vi "Experiment02.vi"() -> ()   [LabVIEW 2009]
uses:
  <vilib>/imath/engines/lvmath2/RunTimeEngine/ErrorHandling/NIMS_Finalize Error.vi
  <vilib>/imath/engines/lvmath2/RunTimeEngine/Parser/MC_Version.vi
  <vilib>/imath/engines/lvmath2/RunTimeEngine/NodeEndStatement/NIMS_NodeEndStatement_Output.vi
  <instcachedir>/0/NIMS_NodeEndStatement_Output_B70DDD75627E4997AAE11E9955EDAA25.lvgen/NIMS_NodeEndStatement_Output_B70DDD75627E4997AAE11E9955EDAA25_003.vi
  <instcachedir>/0/NIMS_NodeEndStatement_Output_B70DDD75627E4997AAE11E9955EDAA25.lvgen/NIMS_NodeEndStatement_Output_B70DDD75627E4997AAE11E9955EDAA25_002.vi
  <vilib>/imath/engines/lvmath/Functions/Error Handling/MergeErrorsWrapper.vi
  <instcachedir>/0/NIMS_NodeEndStatement_Output_B70DDD75627E4997AAE11E9955EDAA25.lvgen/NIMS_NodeEndStatement_Output_B70DDD75627E4997AAE11E9955EDAA25_001.vi
  <vilib>/imath/engines/lvmath2/RunTimeEngine/Managers/WorkSpace/UID Generator.vi
  <vilib>/imath/engines/lvmath/Functions/Error Handling/error.ctl
  <instcachedir>/0/NIMS_NodeEndStatement_Output_B70DDD75627E4997AAE11E9955EDAA25.lvgen/NIMS_NodeEndStatement_Output_B70DDD75627E4997AAE11E9955EDAA25_000.vi
  <vilib>/imath/engines/lvmath2/RunTimeEngine/Managers/SymbolTable/Clear UID.vi
  <vilib>/imath/engines/lvmath2/RunTimeEngine/VariableToken/NIMS_VariableToken_CondDefined.vi
  <instcachedir>/0/NIMS_VariableToken_CondDefined_5641E79000FB4D628475532441475385.lvgen/NIMS_VariableToken_CondDefined_5641E79000FB4D628475532441475385_001.vi
  <vilib>/imath/engines/lvmath/Functions/Error Handling/MC_Mask_Errors.vi
  <vilib>/imath/engines/lvmath2/RunTimeEngine/BuiltInFunctions/rem/NIMS_rem_no checks.vi
  <instcachedir>/0/NIMS_rem_no checks_4CC9B305AB7E42EF90AFC4973FB32F8D.lvgen/NIMS_rem_no checks_4CC9B305AB7E42EF90AFC4973FB32F8D_000.vi
  <vilib>/imath/engines/lvmath2/RunTimeEngine/BuiltInFunctions/uint32/NIMS_uint32(real).vi
  <instcachedir>/0/NIMS_uint32(real)_FDC83D68D45943DDB8F3F934FF8A712F.lvgen/NIMS_uint32(real)_FDC83D68D45943DDB8F3F934FF8A712F_000.vi
  <vilib>/imath/engines/lvmath2/RunTimeEngine/BuiltInFunctions/double/NIMS_double.vi
  <instcachedir>/0/NIMS_double_2CE444F3CE4146B199A482FE12545E45.lvgen/NIMS_double_2CE444F3CE4146B199A482FE12545E45_000.vi
  <vilib>/imath/engines/lvmath2/RunTimeEngine/RangeToken/NIMS_Range.vi
  <instcachedir>/0/NIMS_Range_6D647EC16A744C98B5DE1D649A2D648D.lvgen/NIMS_Range_6D647EC16A744C98B5DE1D649A2D648D_001.vi
  <vilib>/imath/engines/lvmath2/RunTimeEngine/BuiltInFunctions/length/NIMS_length(GV).vi
  <instcachedir>/0/NIMS_length(GV)_7D6E94E728E145E68721C53861296D96.lvgen/NIMS_length(GV)_7D6E94E728E145E68721C53861296D96_000.vi
  <instcachedir>/0/NIMS_Range_6D647EC16A744C98B5DE1D649A2D648D.lvgen/NIMS_Range_6D647EC16A744C98B5DE1D649A2D648D_000.vi
  <vilib>/imathl/engines/lvmath/Functions/Error Handling/Create Error.vi
  <vilib>/imath/engines/lvmath2/RunTimeEngine/ReplaceToken/NIMS_Replace - V(S)=S.vi
  <instcachedir>/0/NIMS_Replace - V(S)=S_670A9E0533664C1D848C8E58B3321B6A.lvgen/NIMS_Replace - V(S)=S_670A9E0533664C1D848C8E58B3321B6A_002.vi
  <vilib>/imath/engines/lvmath2/RunTimeEngine/ReplaceToken/NIMS_Replace - Size Check _(_)=S.vi
  <instcachedir>/0/NIMS_Replace - Size Check _(_)=S_8596181D73404097BAB9CBB006194BB0.lvgen/NIMS_Replace - Size Check _(_)=S_8596181D73404097BAB9CBB006194BB0_002.vi
  <vilib>/imath/engines/lvmath2/RunTimeEngine/ReplaceToken/NIMS_Replace - Check Linear.vi
  <instcachedir>/0/NIMS_Replace - Check Linear_9243CBB174894FF6977027453DA6955E.lvgen/NIMS_Replace - Check Linear_9243CBB174894FF6977027453DA6955E_002.vi
  <vilib>/imath/engines/lvmath2/RunTimeEngine/VariableToken/NIMS_VariableToken_CondDefinedDefinedByReplace.vi
  <instcachedir>/0/NIMS_VariableToken_CondDefinedDefinedByReplace_D162CFFC24174562A9FEA619A91E1A56.lvgen/NIMS_VariableToken_CondDefinedDefinedByReplace_D162CFFC24174562A9FEA619A91E1A56_002.vi
  <vilib>/imath/engines/lvmath2/RunTimeEngine/CommandStatement/MC_CommandStatement_break.vi
  <vilib>/imath/engines/lvmath2/RunTimeEngine/LocalVariableDefStatement/MC_LocalVariableDefStatement_Display.vi
  <vilib>/imath/engines/lvmath2/RunTimeEngine/RunTimeType/NIMS_RunTimeType_From StrictType (excl LVString).vi
  <vilib>/imath/engines/lvmath2/RunTimeEngine/ArithmeticOperatorToken/NIMS_ArithmeticOperator_times.vi
  <instcachedir>/0/NIMS_ArithmeticOperator_times_3987BC660D7947CD8628C10658A43225.lvgen/NIMS_ArithmeticOperator_times_3987BC660D7947CD8628C10658A43225_001.vi
  <instcachedir>/0/NIMS_ArithmeticOperator_times_3987BC660D7947CD8628C10658A43225.lvgen/NIMS_ArithmeticOperator_times_3987BC660D7947CD8628C10658A43225_000.vi
  <vilib>/imath/engines/lvmath2/RunTimeEngine/VariableToken/Read/NIMS_Get Elements - RV(_) - Check.vi
  <instcachedir>/0/NIMS_Get Elements - RV(_) - Check_60F12861D0564803969A5D0D0D1716CD.lvgen/NIMS_Get Elements - RV(_) - Check_60F12861D0564803969A5D0D0D1716CD_000.vi
  <instcachedir>/0/NIMS_VariableToken_CondDefined_5641E79000FB4D628475532441475385.lvgen/NIMS_VariableToken_CondDefined_5641E79000FB4D628475532441475385_000.vi
  <vilib>/imath/engines/lvmath2/RunTimeEngine/BuiltInFunctions/abs/NIMS_abs(signed).vi
  <instcachedir>/0/NIMS_abs(signed)_C4FCB8E6058B49B797C7C8D53CA5F6EC.lvgen/NIMS_abs(signed)_C4FCB8E6058B49B797C7C8D53CA5F6EC_000.vi
  <instcachedir>/0/NIMS_Replace - V(S)=S_670A9E0533664C1D848C8E58B3321B6A.lvgen/NIMS_Replace - V(S)=S_670A9E0533664C1D848C8E58B3321B6A_001.vi
  <instcachedir>/0/NIMS_Replace - Size Check _(_)=S_8596181D73404097BAB9CBB006194BB0.lvgen/NIMS_Replace - Size Check _(_)=S_8596181D73404097BAB9CBB006194BB0_001.vi
  <instcachedir>/0/NIMS_Replace - Check Linear_9243CBB174894FF6977027453DA6955E.lvgen/NIMS_Replace - Check Linear_9243CBB174894FF6977027453DA6955E_001.vi
  <instcachedir>/0/NIMS_VariableToken_CondDefinedDefinedByReplace_D162CFFC24174562A9FEA619A91E1A56.lvgen/NIMS_VariableToken_CondDefinedDefinedByReplace_D162CFFC24174562A9FEA619A91E1A56_001.vi
  <instcachedir>/0/NIMS_Replace - V(S)=S_670A9E0533664C1D848C8E58B3321B6A.lvgen/NIMS_Replace - V(S)=S_670A9E0533664C1D848C8E58B3321B6A_000.vi
  <instcachedir>/0/NIMS_Replace - Size Check _(_)=S_8596181D73404097BAB9CBB006194BB0.lvgen/NIMS_Replace - Size Check _(_)=S_8596181D73404097BAB9CBB006194BB0_000.vi
  <instcachedir>/0/NIMS_Replace - Check Linear_9243CBB174894FF6977027453DA6955E.lvgen/NIMS_Replace - Check Linear_9243CBB174894FF6977027453DA6955E_000.vi
  <instcachedir>/0/NIMS_VariableToken_CondDefinedDefinedByReplace_D162CFFC24174562A9FEA619A91E1A56.lvgen/NIMS_VariableToken_CondDefinedDefinedByReplace_D162CFFC24174562A9FEA619A91E1A56_000.vi
  <vilib>/imath/engines/lvmath2/RunTimeEngine/BuiltInFunctions/imag/NIMS_imag(Complex).vi
  <instcachedir>/0/NIMS_imag(Complex)_D35A2F120E254B34824E500A22AD8EA0.lvgen/NIMS_imag(Complex)_D35A2F120E254B34824E500A22AD8EA0_000.vi
  <vilib>/imath/engines/lvmath2/RunTimeEngine/Managers/SymbolTable/NIMS_WorkSpace.lvlib
panel:
  out "Current VI path 12":string
  out "New Path for Picture 12":string
  out "Part Stripped 12":string
  out "Stripped Path 12":string
  out "Current VI path 11":string
  out "New Path for Picture 11":string
  out "Part Stripped 11":string
  out "Stripped Path 11":string
  out "Current VI path 10":string
  out "New Path for Picture 10":string
  out "Part Stripped 10":string
  out "Stripped Path 10":string
  out "Current VI path 9":string
  out "New Path for Picture 9":string
  out "Part Stripped 9":string
  out "Stripped Path 9":string
  out "Current VI path 8":string
  out "New Path for Picture 8":string
  out "Part Stripped 8":string
  out "Stripped Path 8":string
  out "Current VI path 7":string
  out "New Path for Picture 7":string
  out "Part Stripped 7":string
  out "Stripped Path 7":string
  out "Current VI path 6":string
  out "New Path for Picture 6":string
  out "Part Stripped 6":string
  out "Stripped Path 6":string
  out "Current VI path 5":string
  out "New Path for Picture 5":string
  out "Part Stripped 5":string
  out "Stripped Path 5":string
  out "Current VI path 4":string
  out "New Path for Picture 4":string
  out "Part Stripped 4":string
  out "Stripped Path 4":string
  out "Current VI path 3":string
  out "New Path for Picture 3":string
  out "Part Stripped 3":string
  out "Stripped Path 3":string
  out "Current VI path 2":string
  out "New Path for Picture 2":string
  out "Part Stripped 2":string
  out "Stripped Path 2":string
  out "Current VI path":string
  out "New Path for Picture":string
  out "Part Stripped":string
  out "Stripped Path":string
  out "error out":errorcluster
  in  "HELP FOR VSWR":bool
  out "error out":errorcluster
  out "?":errorcluster
  in  "VSWR Value of Unknown Impedance":bool
  out "?":errorcluster
  out "VSWR Meter":dbl(knob) caption="Meter" scale=500.0..1.0 scale format="%#_10g"
  in  "?":enum32{"LOADS"}(tab)
  in  "Type of Loads":T1(radio)
  out "Resistance 2":dbl
  out "Reactance":dbl
  in  "Resistance":dbl(slide) scale=0.0..1000.0
  in  "Reluctance":dbl(slide) scale=0.0..1000.0
  out "?":errorcluster
  in  "HELP FOR LOADS":bool
  out "error out":errorcluster
  in  "?":enum32{"SLOTTED LINE(VOLTAGE)"}(tab)
  out "?":dbl[](graph)
  in  "Slide":dbl(slide) scale=0.0..0.3
  out "Voltage":dbl
  out "Distance(Meter)":dbl
  out "Characteristic Impedance":dbl
  in  "Short Circuited              Load":bool
  out "?":errorcluster
  in  "First Minima from Load(Unknown Impedance)":bool
  out "?":dbl
  in  "First Minima from Load(Short Circuited)":bool
  in  "Second Minima from Load(Short Circuited)":bool
  out "?":dbl
  in  "HELP FOR SLOTTED LINE":bool
  out "?":dbl
  in  "?":enum32{"ATTENUATOR"}(tab)
  out "?":dbl[](graph)
  in  "Set the value of attenuation in dB":dbl(slide) scale=0.0..100.0
  out "?":errorcluster
  in  "HELP FOR ATTENUATOR":bool
  out "error out":errorcluster
  in  "?":enum32{"ISOLATOR"}(tab)
  out "?":dbl[](graph)
  in  "?":bool
  out "?":errorcluster
  in  "HELP FOR ISOLATOR":bool
  out "error out":errorcluster
  in  "?":enum32{"MODULATOR"}(tab)
  out "?":dbl[](graph)
  in  "Modulating Frequency(KHz)":dbl(slide) scale=0.5..1.5
  out "?":errorcluster
  in  "HELP FOR MODULATOR":bool
  out "error out":errorcluster
  in  "?":enum32{"SOURCE"}(tab)
  out "?":dbl[](graph)
  in  "Frequency of carrier wave(GHz)":dbl(slide) scale=8.0..15.0
  in  "Voltage 3":dbl(knob) scale=0.0..20.0 scale format="%#_10g"
  out "?":errorcluster
  in  "HELP FOR SOURCE":bool
  out "error out":errorcluster
  out "?":errorcluster
  out "Reactance of Unknown Impedance":dbl
  out "Resistance of Unknown Impedance":dbl
  in  "Value of Unknown Impedance":bool
  # "Backward Direction"
  # "Forward direction"
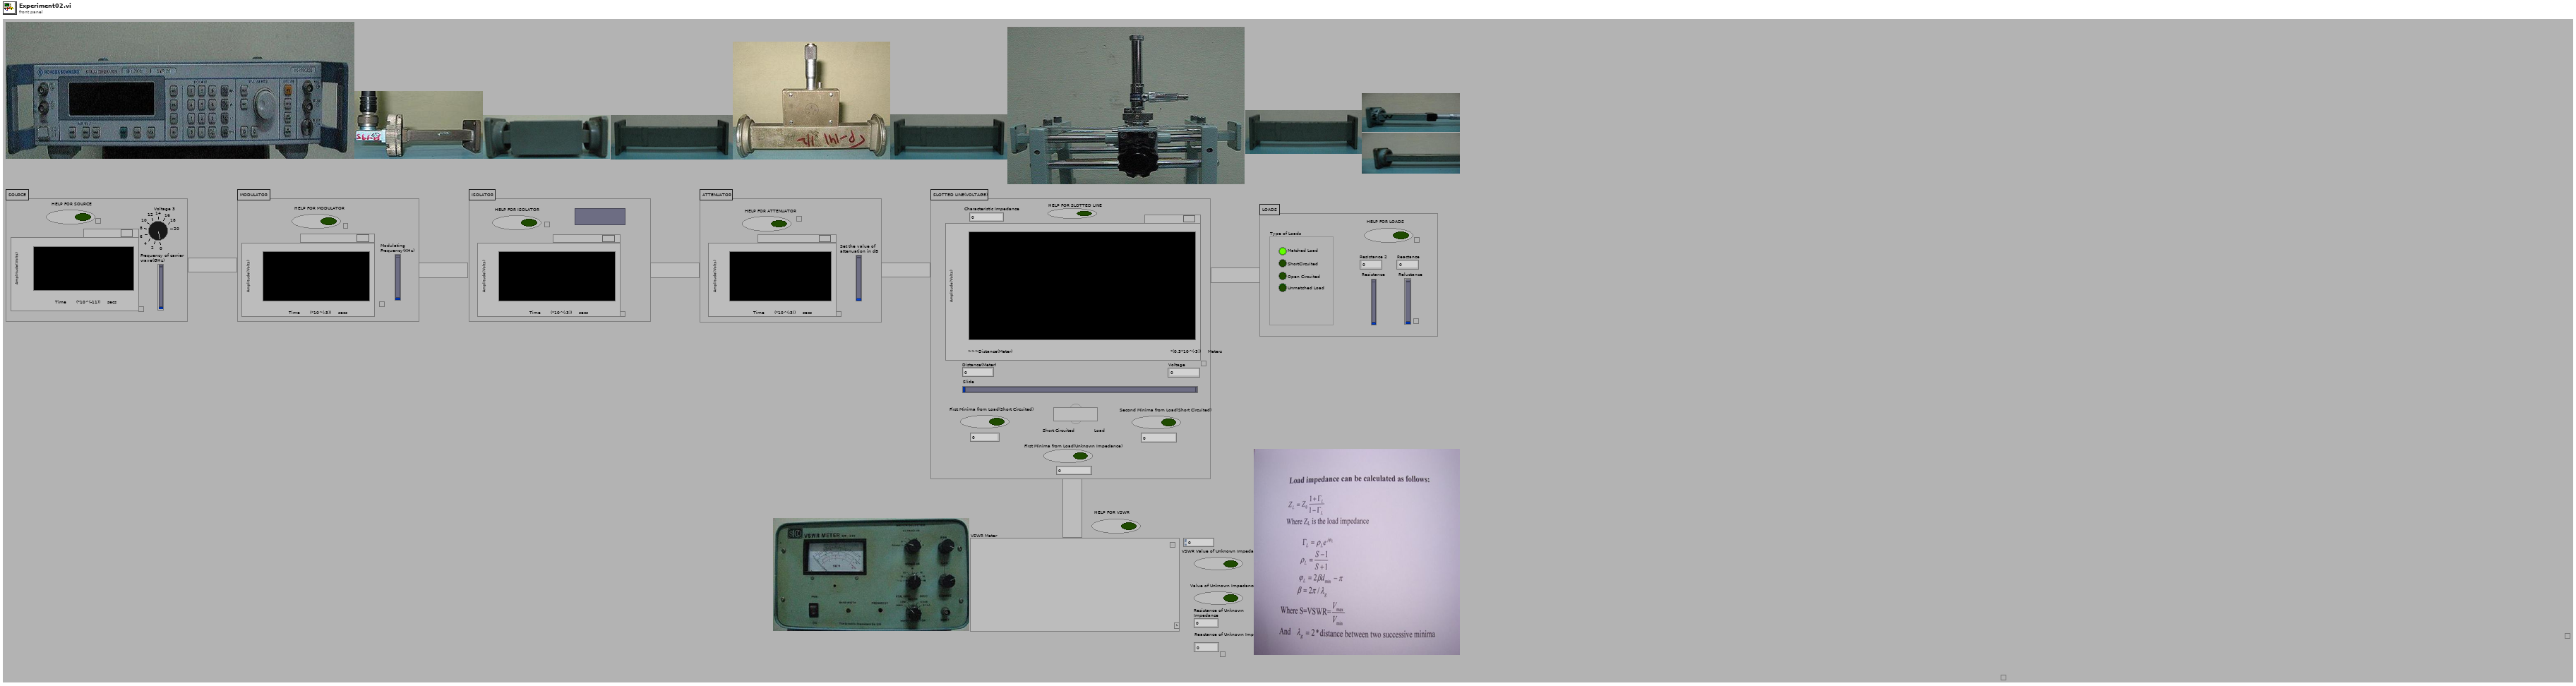
[diagram p1: front panel]
types:
  T1 = enum32{"Matched Load", "ShortCircuited", "Open Circuited", "Unmatched Load"}
  T2 = typedef "imagedata.ctl" = cluster{"image type":i32, "image depth":i32, "image":u8[], "mask":u8[], "colors":u32[], "Rectangle":cluster{"left":i16, "top":i16, "right":i16, "bottom":i16}}
  T3 = typedef "error.ctl" = enum16{"No Error", "Problem", "Unused002", "Incorrect number of parameters", "Function not defined for non-numeric types", "Unused005", "Function only defined for character arrays", "Function not defined for boolean, character, or single precision", "Function not defined for complex types", "Not a valid operation", "Inputs must be scalar", "Input matrices are not the same size", "Unused012", "Input matrices must be nonnegative integers of the same type", "Arguments must be non-negative integers less than bitmax", "Number to complement must be less than 2^N", "Bit to get is outside range", "Bit to set is outside range", "Input must be real type ", "At least one parameter must be scalar", "Unused020", "Function not defined for\nhigher dimensional matrices.", "Invalid attributes", "Wrong Type of Input Arguments", "Wrong Argument Option", "Unused025", "Indices must be real positive integers", "Unused027", "Number of elements must be the same for indices and values", "Unused029", "Cannot resize a 2D matrix with a linear index", "Unknown variable or symbol", "Indices out of range", "Empty matrix deletion can not be used with two indices", "Number of rows and columns must be the same for indices and values.", "Complex cannot be converted to Boolean", "Char cannot be converted to Boolean", "int64 cannot be converted to Boolean", "uint64 cannot be converted to Boolean", "Unused039", "Unused040", "All rows must have the same number of columns", "Incompatible types", "Invalid matrix dimensions", "Dimension must be 1 or 2", "Base must be an integer between 2 and 36", "Invalid input", "Square matrix required", "Function 'timerstart' must be called before 'timerstop'", "Arguments must be positive real", "Step must not be zero", "Wrong number of input arguments", "Wrong number of output arguments", "Unused053", "Input scalar must be >= 0", "Input scalar must be positive", "Input scalar must not be 0", "Input scalar must be in range [0,1]", "Unused058", "Input must be a vector", "Unused060", "Empty vector error", "All elements must be in domain [-1,1]", "All real elements of input vector must be >= 0", "All elements of input vector must be positive", "Values of input vectors are not compatible", "Unused066", "Input vector must be an increasing vector", "Unused068", "Unused069", "Lenths of two input vectors are not compatible", "Unused071", "Empty matrix error", "Unused073", "Unused074", "Unused075", "Unused076", "Unused077", "Size of input matrix is incompatible with input size", "Invalid format specifier", "Unused080", "Unused081", "Unused082", "Unused083", "Unused084", "Unused085", "RunTime: MathScript could not be compiled", "Unknown function", "Only scalars and strings supported", "Unused089", "Unused090", "Range is too large", "End used without variable", "Function not available (RTE)", "Custom user error", "Arguments must be integers less than bitmax", "Shared library not found", "Header file not found", "Shared library already loaded", "Shared library not loaded", "Shared library function not found", "Shared library string return problem", "Problem calling shared library function", "Problem loading shared library from OS", "Problem parsing shared library header file", "Shared library incompatible types", "Shared library unsupported return type", "Shared library function not exported", "Shared library unsupported input type", "Problem unloading shared library from OS", "Function only available from UI", "Invalid function specified in argument", "An internal error has occurred", "Invalid object", "Invalid property", "Read-only property", "A break command has occurred", "A continue command has occurred", "A return command has occurred", "ode: times parameter invalid", "Unused120", "Function not found in file", "Reserved keyword cannot be defined as variable", "Reserved keyword cannot be defined as a function or script", "Arguments must be string literals", "Function not supported on this platform", "All columns must have the same number of rows", "Function ignored in RTE warning", "Cannot use : as a parameter that is not a variable", "Output can't be coerced to requested type", "Function not supported on current target", "Variable dependent on an unwired function input", "Unused132", "Unused133", "Unused134", "Unused135", "Unused136", "Unused137", "Unused138", "Unused139", "Unused140", "Unused141", "Unused142", "Unused143", "Unused144", "Unused145", "Unused146", "MathScript parser DLL missing", "MathScript requires LabVIEW Full", "MathScript license is invalid or missing"}
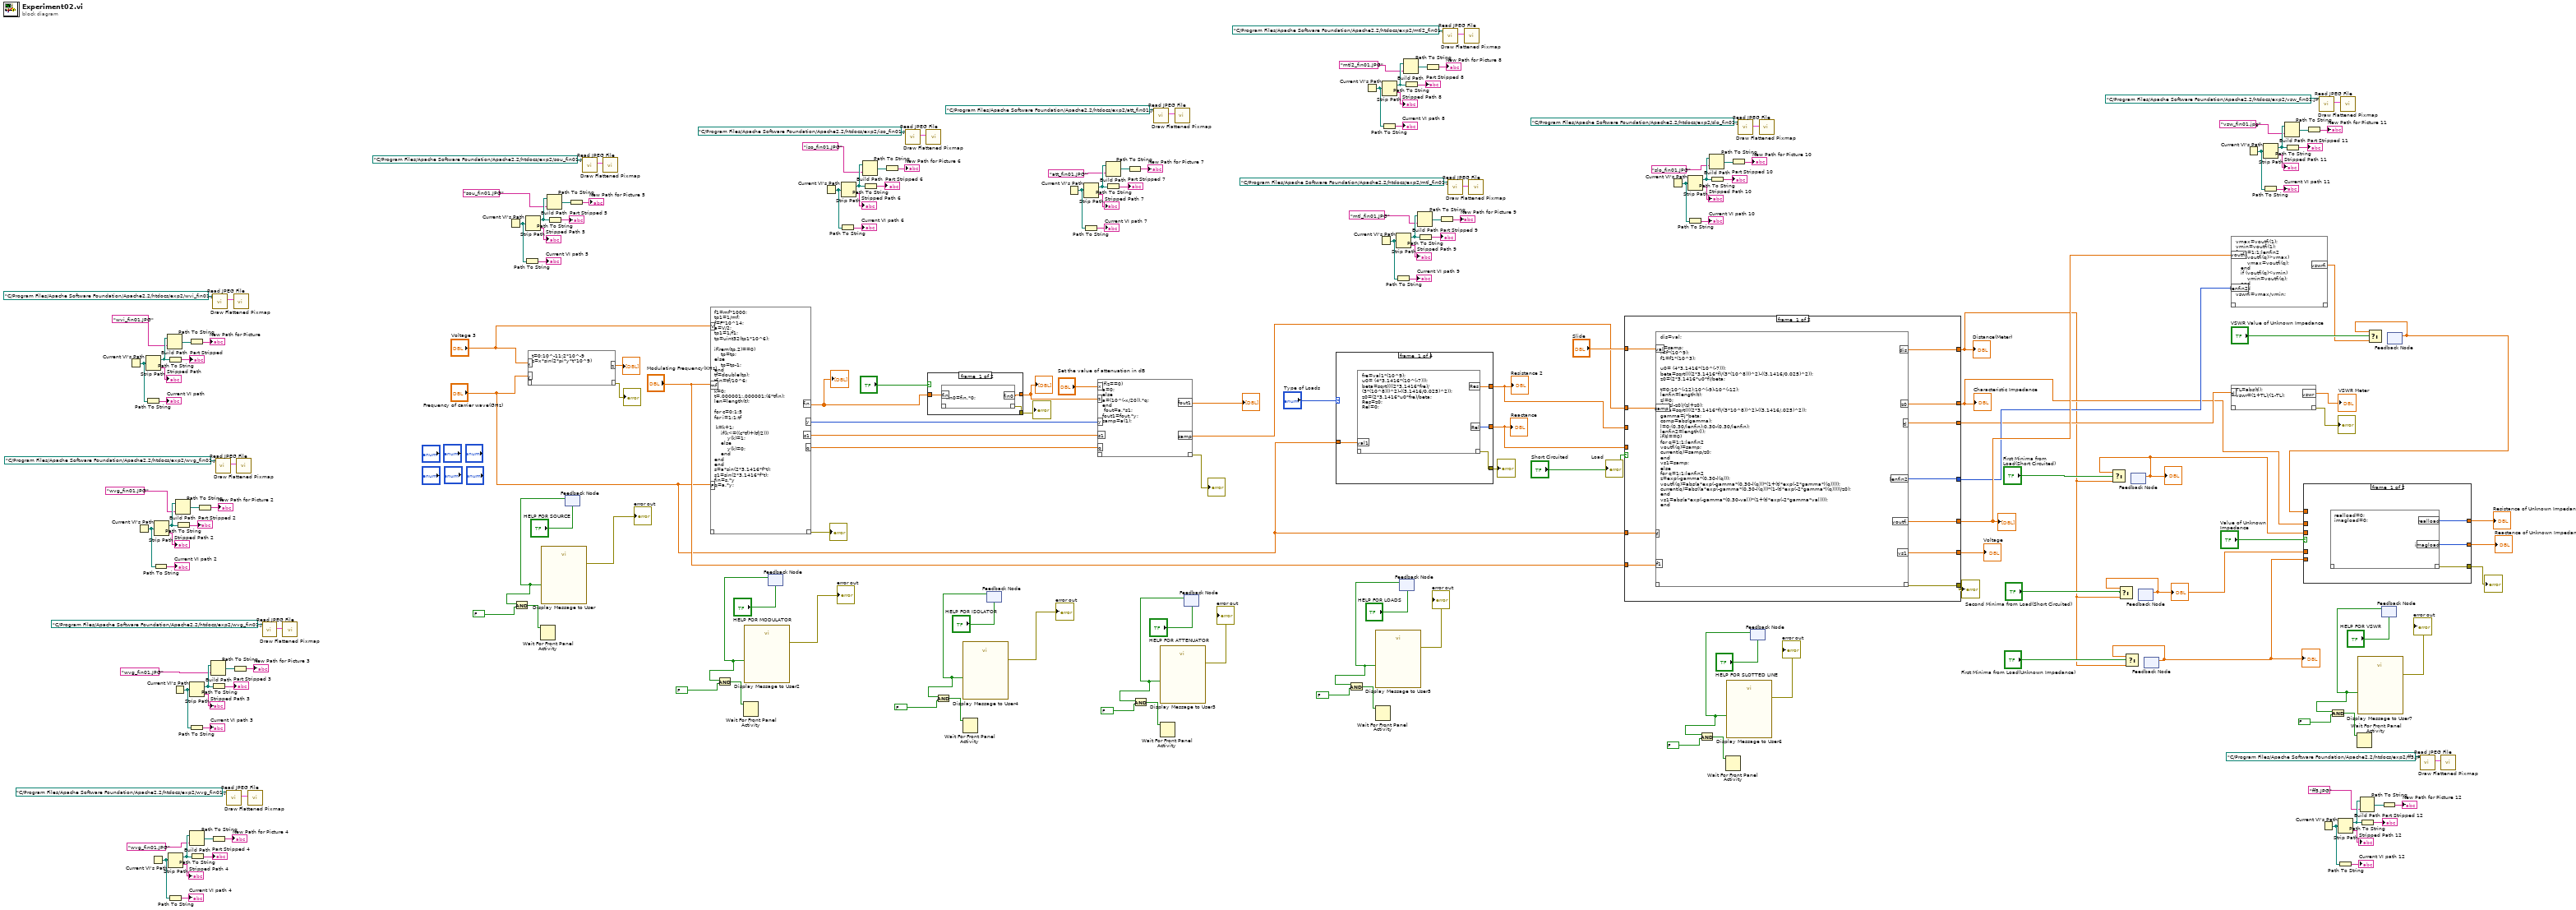
[diagram p0: block diagram]
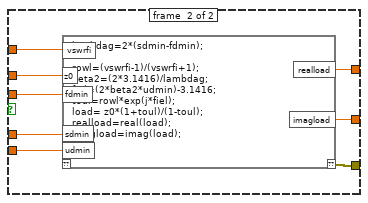
[diagram p2: hidden frame]
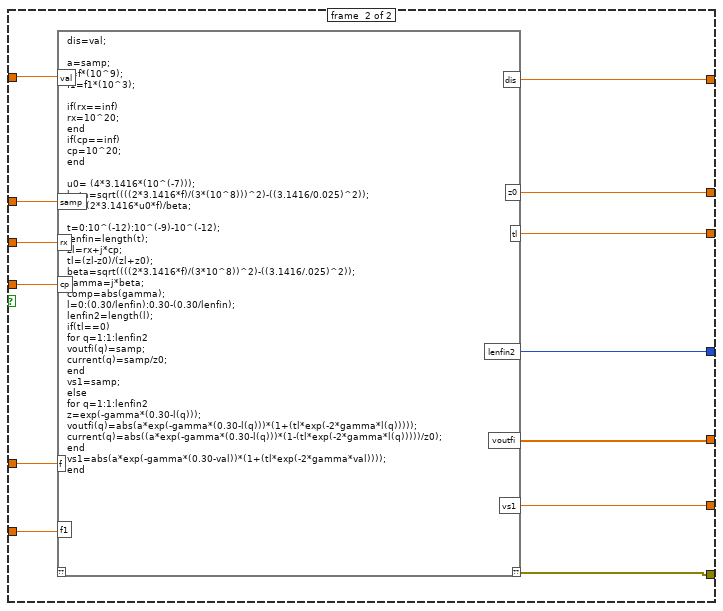
[diagram p3: hidden frame]
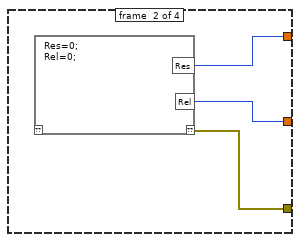
[diagram p4: hidden frame]
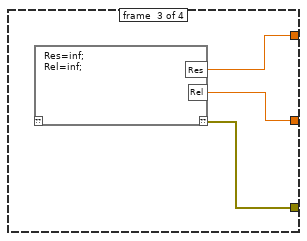
[diagram p5: hidden frame]
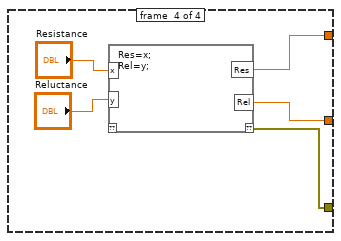
[diagram p6: hidden frame]
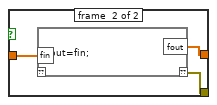
[diagram p7: hidden frame]
diagram:
  n1 = Current VI's Path() -> (path=w103:path)
  n2 = Current VI's Path() -> (path=w95:path)
  n3 = Path To String(path=w103) -> (string=→"Current VI path":string)
  n4 = Strip Path(path=w103) -> (stripped path=w108:path, name=→"Stripped Path":string)
  n5 = Current VI's Path() -> (path=w79:path)
  n6 = Path To String(path=w95) -> (string=→"Current VI path 2":string)
  n7 = Strip Path(path=w95) -> (stripped path=w100:path, name=→"Stripped Path 2":string)
  n8 = Build Path(base path=w108, name or relative path="wvi_fin01.JPG") -> (appended path=w101:path)
  n9 = Path To String(path=w108) -> (string=→"Part Stripped":string)
  n10 = Path To String(path=w79) -> (string=→"Current VI path 4":string)
  n11 = Strip Path(path=w79) -> (stripped path=w84:path, name=→"Stripped Path 4":string)
  n12 = Current VI's Path() -> (path=w87:path)
  n13 = Build Path(base path=w100, name or relative path="wvg_fin01.JPG") -> (appended path=w93:path)
  n14 = Path To String(path=w100) -> (string=→"Part Stripped 2":string)
  n15 = Path To String(path=w101) -> (string=→"New Path for Picture":string)
  n16 = Path To String(path=w87) -> (string=→"Current VI path 3":string)
  n17 = Strip Path(path=w87) -> (stripped path=w92:path, name=→"Stripped Path 3":string)
  n18 = Build Path(base path=w84, name or relative path="wvg_fin01.JPG") -> (appended path=w77:path)
  n19 = Path To String(path=w84) -> (string=→"Part Stripped 4":string)
  n20 = Path To String(path=w93) -> (string=→"New Path for Picture 2":string)
  n21 = Build Path(base path=w92, name or relative path="wvg_fin01.JPG") -> (appended path=w85:path)
  n22 = Path To String(path=w92) -> (string=→"Part Stripped 3":string)
  n23 = Path To String(path=w77) -> (string=→"New Path for Picture 4":string)
  n24 = call <vilib>:"Read JPEG File.vi"("path to JPEG file"=path "C:/Program Files/Apache Software Foundation/Apache2.2/htdocs/exp2/wvi_fin01.JPG") -> ("image data"=w118:T2)  [unwired: 1 in, 9 out]
  n25 = call <vilib>:"Read JPEG File.vi"("path to JPEG file"=path "C:/Program Files/Apache Software Foundation/Apache2.2/htdocs/exp2/wvg_fin01.JPG") -> ("image data"=w116:T2)  [unwired: 1 in, 9 out]
  n26 = call <vilib>:"Read JPEG File.vi"("path to JPEG file"=path "C:/Program Files/Apache Software Foundation/Apache2.2/htdocs/exp2/wvg_fin01.JPG") -> ("image data"=w112:T2)  [unwired: 1 in, 9 out]
  n27 = Path To String(path=w85) -> (string=→"New Path for Picture 3":string)
  n28 = call <vilib>:"Draw Flattened Pixmap.vi"("image data"=w118) -> ()  [unwired: 1 in, 8 out]
  n29 = call <vilib>:"Draw Flattened Pixmap.vi"("image data"=w116) -> ()  [unwired: 1 in, 8 out]
  n30 = call <vilib>:"Draw Flattened Pixmap.vi"("image data"=w112) -> ()  [unwired: 1 in, 8 out]
  n31 = call <vilib>:"Read JPEG File.vi"("path to JPEG file"=path "C:/Program Files/Apache Software Foundation/Apache2.2/htdocs/exp2/wvg_fin01.JPG") -> ("image data"=w113:T2)  [unwired: 1 in, 9 out]
  n32 = call <vilib>:"Draw Flattened Pixmap.vi"("image data"=w113) -> ()  [unwired: 1 in, 8 out]
  n33 = Current VI's Path() -> (path=w71:path)
  n34 = Path To String(path=w71) -> (string=→"Current VI path 5":string)
  n35 = Strip Path(path=w71) -> (stripped path=w76:path, name=→"Stripped Path 5":string)
  n36 = mathscript code="t=0:10^-11:2*10^-9\nz=x*sin(2*pi*y*t*10^9)"("x"="Voltage 3", "y"="Frequency of carrier wave(GHz)") -> ("??"=→"?":errorcluster, "z"=→"?":dbl[])  [unwired: 1 in]
  n37 = Build Path(base path=w76, name or relative path="sou_fin01.JPG") -> (appended path=w69:path)
  n38 = Path To String(path=w76) -> (string=→"Part Stripped 5":string)
  n39 = feedback #1("HELP FOR SOURCE") -> (w195:bool)
  n40 = And(x=w195, y=FALSE) -> (x .and. y?=w193:bool)
  n41 = Wait For Front Panel Activity(3:w193) -> ()  [unwired: 3 out]
  n42 = call "Display Message to User"("Enable"=w195) -> ("error out"=→"error out":errorcluster, "CLOSE"=w197:bool)  [unwired: 2 in, 7 out]
  n43 = Path To String(path=w69) -> (string=→"New Path for Picture 5":string)
  n44 = call <vilib>:"Read JPEG File.vi"("path to JPEG file"=path "C:/Program Files/Apache Software Foundation/Apache2.2/htdocs/exp2/sou_fin01.JPG") -> ("image data"=w119:T2)  [unwired: 1 in, 9 out]
  n45 = call <vilib>:"Draw Flattened Pixmap.vi"("image data"=w119) -> ()  [unwired: 1 in, 8 out]
  n46 = mathscript code="f1=mf*1000;\ntp1=1/mf;\nf=F*10^14;\na=V/2;\ntp1=1/f1;\ntp=uint32(tp1*10^6);\n\nif(rem(tp,2)==0)\n    tp=tp;\nelse\n    tp=tp-1;\nend\ntf=double(tp);\ntfin=tf/10^6;\n\nk=0;\nt=.000001:.000001:(6*tfin);\nlen=length(t);\n\nfor c=0:1:5\nfor i=1:1:tf\n  \n k=k+1;\n    if(k<=((c*tf)+(tf/2)))\n        y(k)=1;\n    else\n        y(k)=0;\n    end\nend\nend\ns=a*sin(2*3.1416*f*t);\ns1=sin(2*3.1416*f*t);\nfin=s.*y\nq=a.*y;"("V"="Voltage 3", "mf"="Modulating Frequency(KHz)", "F"="Frequency of carrier wave(GHz)") -> ("??"=→"?":errorcluster, "fin"=w150:dbl[], "y"=w146:i32[], "s1"=w145:dbl[], "q"=w144:dbl[])  [unwired: 1 in]
  "?" <- w150
  n47 = feedback #2("HELP FOR MODULATOR") -> (w189:bool)
  n48 = And(x=w189, y=FALSE) -> (x .and. y?=w187:bool)
  n49 = Wait For Front Panel Activity(3:w187) -> ()  [unwired: 3 out]
  n50 = call "Display Message to User2"("Enable"=w189) -> ("error out"=→"error out":errorcluster, "CLOSE"=w191:bool)  [unwired: 2 in, 7 out]
  n51 = Current VI's Path() -> (path=w63:path)
  n52 = Path To String(path=w63) -> (string=→"Current VI path 6":string)
  n53 = Strip Path(path=w63) -> (stripped path=w68:path, name=→"Stripped Path 6":string)
  n54 = Build Path(base path=w68, name or relative path="iso_fin01.JPG") -> (appended path=w61:path)
  n55 = Path To String(path=w68) -> (string=→"Part Stripped 6":string)
  n56 = Path To String(path=w61) -> (string=→"New Path for Picture 6":string)
  n57 = call <vilib>:"Read JPEG File.vi"("path to JPEG file"=path "C:/Program Files/Apache Software Foundation/Apache2.2/htdocs/exp2/iso_fin01.JPG") -> ("image data"=w117:T2)  [unwired: 1 in, 9 out]
  n58 = call <vilib>:"Draw Flattened Pixmap.vi"("image data"=w117) -> ()  [unwired: 1 in, 8 out]
  n59 = case shown="False" "?" {
    tunnel: w150 -> [w214 w235]
    tunnel: [w212 w234] -> w207
    tunnel: [w213 w233] -> w147
    frame #0 {
      n60 = mathscript code="fin0=fin.*0;"("fin"=w214) -> ("??"=w212:errorcluster, "fin0"=w213:dbl[])  [unwired: 1 in]
    }
    frame #1 {
      n61 = mathscript code="fout=fin;"("fin"=w235) -> ("??"=w234:errorcluster, "fout"=w233:dbl[])  [unwired: 1 in]
    }
  }
  "?" <- w147
  "?" <- w207
  n62 = feedback #3("HELP FOR ISOLATOR") -> (w177:bool)
  n63 = And(x=w177, y=FALSE) -> (x .and. y?=w175:bool)
  n64 = Wait For Front Panel Activity(3:w175) -> ()  [unwired: 3 out]
  n65 = call "Display Message to User4"("Enable"=w177) -> ("error out"=→"error out":errorcluster, "CLOSE"=w179:bool)  [unwired: 2 in, 7 out]
  n66 = Current VI's Path() -> (path=w55:path)
  n67 = Path To String(path=w55) -> (string=→"Current VI path 7":string)
  n68 = Strip Path(path=w55) -> (stripped path=w60:path, name=→"Stripped Path 7":string)
  n69 = mathscript code="if(z==0)\na=0; \nelse\na=(10^(-x/20)).*q;\nend\n fout=a.*s1;\nfout1=fout.*y;\nsamp=a(1);"("x"="Set the value of attenuation in dB", "z"=w147, "y"=w146, "s1"=w145, "q"=w144) -> ("??"=→"?":errorcluster, "fout1"=→"?":dbl[], "samp"=w141:dbl)  [unwired: 1 in]
  n70 = Build Path(base path=w60, name or relative path="att_fin01.JPG") -> (appended path=w53:path)
  n71 = Path To String(path=w60) -> (string=→"Part Stripped 7":string)
  n72 = Path To String(path=w53) -> (string=→"New Path for Picture 7":string)
  n73 = call <vilib>:"Read JPEG File.vi"("path to JPEG file"=path "C:/Program Files/Apache Software Foundation/Apache2.2/htdocs/exp2/att_fin01.JPG") -> ("image data"=w115:T2)  [unwired: 1 in, 9 out]
  n74 = call <vilib>:"Draw Flattened Pixmap.vi"("image data"=w115) -> ()  [unwired: 1 in, 8 out]
  n75 = feedback #4("HELP FOR ATTENUATOR") -> (w183:bool)
  n76 = And(x=w183, y=FALSE) -> (x .and. y?=w181:bool)
  n77 = Wait For Front Panel Activity(3:w181) -> ()  [unwired: 3 out]
  n78 = call "Display Message to User3"("Enable"=w183) -> ("error out"=→"error out":errorcluster, "CLOSE"=w185:bool)  [unwired: 2 in, 7 out]
  n79 = case shown="\"Unmatched Load\"" "Type of Loads" {
    tunnel: "Frequency of carrier wave(GHz)" -> [w255 _ _ _]
    tunnel: [w252 w341 w368 w394] -> w209
    tunnel: [w253 w340 w367 w393] -> w208
    tunnel: [w254 w342 w366 w392] -> w206
    frame #0 {
      n80 = mathscript code="fre=val1*(10^9);\nu0= (4*3.1416*(10^(-7)));\nbeta=sqrt((((2*3.1416*fre)/(3*(10^8)))^2)-((3.1416/0.025)^2));\nz0=(2*3.1416*u0*fre)/beta;\nRes=z0;\nRel=0;"("val1"=w255) -> ("??"=w254:errorcluster, "Res"=w252:cdb, "Rel"=w253:i32)  [unwired: 1 in]
    }
    frame #1 {
      n81 = mathscript code="Res=0;\nRel=0;"() -> ("??"=w342:errorcluster, "Res"=w341:i32, "Rel"=w340:i32)  [unwired: 1 in]
    }
    frame #2 {
      n82 = mathscript code="Res=inf;\nRel=inf;"() -> ("??"=w366:errorcluster, "Res"=w368:dbl, "Rel"=w367:dbl)  [unwired: 1 in]
    }
    frame #3 {
      n83 = mathscript code="Res=x;\nRel=y;"("x"="Resistance", "y"="Reluctance") -> ("??"=w392:errorcluster, "Res"=w394:dbl, "Rel"=w393:dbl)  [unwired: 1 in]
    }
  }
  "Resistance 2" <- w209
  "Reactance" <- w208
  "?" <- w206
  n84 = Current VI's Path() -> (path=w47:path)
  n85 = Current VI's Path() -> (path=w39:path)
  n86 = Path To String(path=w47) -> (string=→"Current VI path 8":string)
  n87 = Strip Path(path=w47) -> (stripped path=w52:path, name=→"Stripped Path 8":string)
  n88 = Path To String(path=w39) -> (string=→"Current VI path 9":string)
  n89 = Strip Path(path=w39) -> (stripped path=w44:path, name=→"Stripped Path 9":string)
  n90 = feedback #5("HELP FOR LOADS") -> (w171:bool)
  n91 = And(x=w171, y=FALSE) -> (x .and. y?=w169:bool)
  n92 = Wait For Front Panel Activity(3:w169) -> ()  [unwired: 3 out]
  n93 = call "Display Message to User5"("Enable"=w171) -> ("error out"=→"error out":errorcluster, "CLOSE"=w173:bool)  [unwired: 2 in, 7 out]
  n94 = Build Path(base path=w52, name or relative path="mtl2_fin01.JPG") -> (appended path=w45:path)
  n95 = Path To String(path=w52) -> (string=→"Part Stripped 8":string)
  n96 = Build Path(base path=w44, name or relative path="mtl_fin01.JPG") -> (appended path=w37:path)
  n97 = Path To String(path=w44) -> (string=→"Part Stripped 9":string)
  n98 = Path To String(path=w45) -> (string=→"New Path for Picture 8":string)
  n99 = Path To String(path=w37) -> (string=→"New Path for Picture 9":string)
  n100 = call <vilib>:"Read JPEG File.vi"("path to JPEG file"=path "C:/Program Files/Apache Software Foundation/Apache2.2/htdocs/exp2/mtl2_fin01.JPG") -> ("image data"=w110:T2)  [unwired: 1 in, 9 out]
  n101 = call <vilib>:"Read JPEG File.vi"("path to JPEG file"=path "C:/Program Files/Apache Software Foundation/Apache2.2/htdocs/exp2/mtl_fin01.JPG") -> ("image data"=w111:T2)  [unwired: 1 in, 9 out]
  n102 = call <vilib>:"Draw Flattened Pixmap.vi"("image data"=w110) -> ()  [unwired: 1 in, 8 out]
  n103 = call <vilib>:"Draw Flattened Pixmap.vi"("image data"=w111) -> ()  [unwired: 1 in, 8 out]
  n104 = case shown="True" "Short Circuited              Load" {
    tunnel: w209 -> [_ w1013]
    tunnel: w208 -> [_ w1012]
    tunnel: [w429 w1008] -> w134
    tunnel: "Frequency of carrier wave(GHz)" -> [w432 w1011]
    tunnel: "Modulating Frequency(KHz)" -> [w431 w1010]
    tunnel: w141 -> [w433 w1014]
    tunnel: [w424 w1003] -> w205
    tunnel: [w426 w1005] -> w140
    tunnel: [w428 w1007] -> w138
    tunnel: "Slide" -> [w434 w1015]
    tunnel: [w425 w1004] -> w202
    tunnel: [w430 w1009] -> w126
    tunnel: [w427 w1006] -> w139
    frame #0 {
      n105 = mathscript code="dis=val;\n\na=samp;\nf=f*(10^9);\nf1=f1*(10^3);\n\nu0= (4*3.1416*(10^(-7)));\nbeta=sqrt((((2*3.1416*f)/(3*(10^8)))^2)-((3.1416/0.025)^2));\nz0=(2*3.1416*u0*f)/beta;\n\nt=0:10^(-12):10^(-9)-10^(-12);\nlenfin=length(t);\nzl=0;\ntl=(zl-z0)/(zl+z0);\nbeta=sqrt((((2*3.1416*f)/(3*10^8))^2)-((3.1416/.025)^2));\ngamma=j*beta;\ncomp=abs(gamma);\nl=0:(0.30/lenfin):0.30-(0.30/lenfin);\nlenfin2=length(l);\nif(tl==0)\nfor q=1:1:lenfin2\nvoutfi(q)=samp;\ncurrent(q)=samp/z0;\nend\nvs1=samp;\nelse\nfor q=1:1:lenfin2\nz=exp(-gamma*(0.30-l(q)));\nvoutfi(q)=abs(a*exp(-gamma*(0.30-l(q)))*(1+(tl*exp(-2*gamma*l(q)))));\ncurrent(q)=abs((a*exp(-gamma*(0.30-l(q)))*(1-(tl*exp(-2*gamma*l(q)))))/z0);\nend\nvs1=abs(a*exp(-gamma*(0.30-val))*(1+(tl*exp(-2*gamma*val))));\nend"("val"=w434, "samp"=w433, "f"=w432, "f1"=w431) -> ("??"=w424:errorcluster, "dis"=w430:dbl, "z0"=w429:cdb, "tl"=w428:cdb, "lenfin2"=w427:i32, "voutfi"=w426:dbl[], "vs1"=w425:dbl)  [unwired: 1 in]
    }
    frame #1 {
      n106 = mathscript code="dis=val;\n\na=samp;\nf=f*(10^9);\nf1=f1*(10^3);\n\nif(rx==inf)\nrx=10^20;\nend\nif(cp==inf)\ncp=10^20;\nend\n\nu0= (4*3.1416*(10^(-7)));\nbeta=sqrt((((2*3.1416*f)/(3*(10^8)))^2)-((3.1416/0.025)^2));\nz0=(2*3.1416*u0*f)/beta;\n\nt=0:10^(-12):10^(-9)-10^(-12);\nlenfin=length(t);\nzl=rx+j*cp;\ntl=(zl-z0)/(zl+z0);\nbeta=sqrt((((2*3.1416*f)/(3*10^8))^2)-((3.1416/.025)^2));\ngamma=j*beta;\ncomp=abs(gamma);\nl=0:(0.30/lenfin):0.30-(0.30/lenfin);\nlenfin2=length(l);\nif(tl==0)\nfor q=1:1:lenfin2\nvoutfi(q)=samp;\ncurrent(q)=samp/z0;\nend\nvs1=samp;\nelse\nfor q=1:1:lenfin2\nz=exp(-gamma*(0.30-l(q)));\nvoutfi(q)=abs(a*exp(-gamma*(0.30-l(q)))*(1+(tl*exp(-2*gamma*l(q)))));\ncurrent(q)=abs((a*exp(-gamma*(0.30-l(q)))*(1-(tl*exp(-2*gamma*l(q)))))/z0);\nend\nvs1=abs(a*exp(-gamma*(0.30-val))*(1+(tl*exp(-2*gamma*val))));\nend"("val"=w1015, "samp"=w1014, "rx"=w1013, "cp"=w1012, "f"=w1011, "f1"=w1010) -> ("??"=w1003:errorcluster, "dis"=w1009:dbl, "z0"=w1008:cdb, "tl"=w1007:cdb, "lenfin2"=w1006:i32, "voutfi"=w1005:dbl[], "vs1"=w1004:dbl)  [unwired: 1 in]
    }
  }
  "?" <- w140
  "Characteristic Impedance" <- w134
  "?" <- w205
  "Voltage" <- w202
  "Distance(Meter)" <- w126
  n107 = Current VI's Path() -> (path=w31:path)
  n108 = Path To String(path=w31) -> (string=→"Current VI path 10":string)
  n109 = Strip Path(path=w31) -> (stripped path=w36:path, name=→"Stripped Path 10":string)
  n110 = Build Path(base path=w36, name or relative path="slo_fin01.JPG") -> (appended path=w29:path)
  n111 = Path To String(path=w36) -> (string=→"Part Stripped 10":string)
  n112 = Path To String(path=w29) -> (string=→"New Path for Picture 10":string)
  n113 = call <vilib>:"Read JPEG File.vi"("path to JPEG file"=path "C:/Program Files/Apache Software Foundation/Apache2.2/htdocs/exp2/slo_fin01.JPG") -> ("image data"=w114:T2)  [unwired: 1 in, 9 out]
  n114 = feedback #6("HELP FOR SLOTTED LINE") -> (w164:bool)
  n115 = And(x=w164, y=FALSE) -> (x .and. y?=w162:bool)
  n116 = Wait For Front Panel Activity(3:w162) -> ()  [unwired: 3 out]
  n117 = call "Display Message to User6"("Enable"=w164) -> ("error out"=→"error out":errorcluster, "CLOSE"=w166:bool)  [unwired: 2 in, 7 out]
  n118 = call <vilib>:"Draw Flattened Pixmap.vi"("image data"=w114) -> ()  [unwired: 1 in, 8 out]
  n119 = feedback #7() -> (w125:dbl)  [unwired: 1 in]
  "?" <- w125
  n120 = Select(t=w125, s="First Minima from Load(Short Circuited)", f=w126) -> (s? t:f=w132:dbl)
  n121 = feedback #8() -> (w130:dbl)  [unwired: 1 in]
  "?" <- w130
  n122 = Select(t=w130, s="Second Minima from Load(Short Circuited)", f=w126) -> (s? t:f=w131:dbl)
  n123 = feedback #9() -> (w124:dbl)  [unwired: 1 in]
  "?" <- w124
  n124 = Select(t=w124, s="First Minima from Load(Unknown Impedance)", f=w126) -> (s? t:f=w128:dbl)
  n125 = mathscript code="vmax=voutfi(1);\nvmin=voutfi(1);\nfor q=1:1:lenfin2\n   if (voutfi(q)>vmax)\n       vmax=voutfi(q);\n   end\n   if (voutfi(q)<vmin)\n       vmin=voutfi(q);\n   end\n   end\nvswrfi=vmax/vmin;"("lenfin2"=w139, "voutfi"=w140) -> ("vswrfi"=w121:dbl)  [unwired: 1 in, 1 out]
  n126 = mathscript code="TL=abs(tl);\nvswr=(1+TL)/(1-TL);"("tl"=w138) -> ("??"=→"?":errorcluster, "vswr"=→"VSWR Meter":dbl)  [unwired: 1 in]
  n127 = Current VI's Path() -> (path=w23:path)
  n128 = Path To String(path=w23) -> (string=→"Current VI path 11":string)
  n129 = Strip Path(path=w23) -> (stripped path=w28:path, name=→"Stripped Path 11":string)
  n130 = Build Path(base path=w28, name or relative path="vsw_fin01.jpg") -> (appended path=w21:path)
  n131 = Path To String(path=w28) -> (string=→"Part Stripped 11":string)
  n132 = Path To String(path=w21) -> (string=→"New Path for Picture 11":string)
  n133 = call <vilib>:"Read JPEG File.vi"("path to JPEG file"=path "C:/Program Files/Apache Software Foundation/Apache2.2/htdocs/exp2/vsw_fin01.JPG") -> ("image data"=w109:T2)  [unwired: 1 in, 9 out]
  n134 = Current VI's Path() -> (path=w15:path)
  n135 = Path To String(path=w15) -> (string=→"Current VI path 12":string)
  n136 = Strip Path(path=w15) -> (stripped path=w20:path, name=→"Stripped Path 12":string)
  n137 = call <vilib>:"Draw Flattened Pixmap.vi"("image data"=w109) -> ()  [unwired: 1 in, 8 out]
  n138 = Build Path(base path=w20, name or relative path="ff5.JPG") -> (appended path=w13:path)
  n139 = Path To String(path=w20) -> (string=→"Part Stripped 12":string)
  n140 = feedback #10("HELP FOR VSWR") -> (w158:bool)
  n141 = And(x=w158, y=FALSE) -> (x .and. y?=w156:bool)
  n142 = Wait For Front Panel Activity(3:w156) -> ()  [unwired: 3 out]
  n143 = call "Display Message to User7"("Enable"=w158) -> ("error out"=→"error out":errorcluster, "CLOSE"=w160:bool)  [unwired: 2 in, 7 out]
  n144 = Path To String(path=w13) -> (string=→"New Path for Picture 12":string)
  n145 = feedback #11() -> (w120:dbl)  [unwired: 1 in]
  n146 = case shown="True" "Value of Unknown Impedance" {
    tunnel: [w1625 w1652] -> w201
    tunnel: [w1624 w1651] -> w200
    tunnel: w130 -> [_ w1654]
    tunnel: w124 -> [_ w1653]
    tunnel: w120 -> [_ w1656]
    tunnel: w134 -> [_ w1655]
    tunnel: [w1623 w1650] -> w135
    tunnel: w125 -> [_ w1649]
    frame #0 {
      n147 = mathscript code="realload=0;\nimagload=0;"() -> ("??"=w1623:errorcluster, "realload"=w1625:i32, "imagload"=w1624:i32)  [unwired: 1 in]
    }
    frame #1 {
      n148 = mathscript code="lambdag=2*(sdmin-fdmin);\n\nrowl=(vswrfi-1)/(vswrfi+1);\nbeta2=(2*3.1416)/lambdag;\nfiel=(2*beta2*udmin)-3.1416;\ntoul=rowl*exp(j*fiel);\nload= z0*(1+toul)/(1-toul);\nrealload=real(load);\nimagload=imag(load);"("vswrfi"=w1656, "z0"=w1655, "fdmin"=w1649, "sdmin"=w1654, "udmin"=w1653) -> ("??"=w1650:errorcluster, "realload"=w1652:dbl, "imagload"=w1651:dbl)  [unwired: 1 in]
    }
  }
  "Resistance of Unknown Impedance" <- w201
  "Reactance of Unknown Impedance" <- w200
  "?" <- w135
  n149 = Select(t=w120, s="VSWR Value of Unknown Impedance", f=w121) -> (s? t:f=w123:dbl)
  n150 = call <vilib>:"Read JPEG File.vi"("path to JPEG file"=path "C:/Program Files/Apache Software Foundation/Apache2.2/htdocs/exp2/ff5.JPG") -> ("image data"=w168:T2)  [unwired: 1 in, 9 out]
  n151 = call <vilib>:"Draw Flattened Pixmap.vi"("image data"=w168) -> ()  [unwired: 1 in, 8 out]
